vi "Close.vi"(8 "error in (no error)":errorcluster, 11 "Query Result in":refnum<class "Query Result.lvclass">) -> (0 "error out":errorcluster)   [LabVIEW 2020, in "ORM.lvlib" / "Query Result.lvclass"]
uses:
  Query Result.lvclass
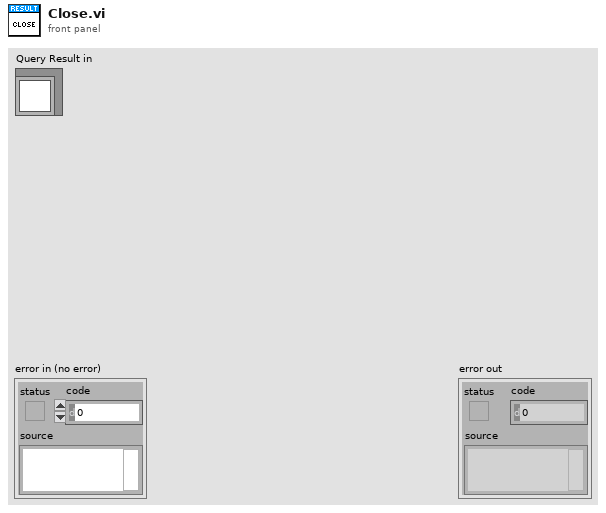
[diagram p1: front panel]
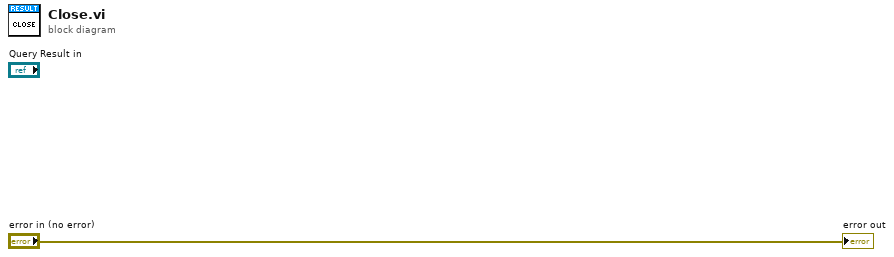
[diagram p0: block diagram]
diagram:
  "error out" <- "error in (no error)"
